vi "call service _ get time.vi"(7 "error in (no error)":errorcluster, 10 "TCP Network Connection in":refnum<k5>) -> (0 "error out":errorcluster, 2 "value":T1, 3 "TCP Network Connection out":refnum<k5>)   [LabVIEW 2015]
uses:
  <vilib>/MediaMongrels Ltd/WebSockets/WebSockets/WebSockets.lvlib
panel:
  in  "ros call service ctl.":T1
  out "Data":string
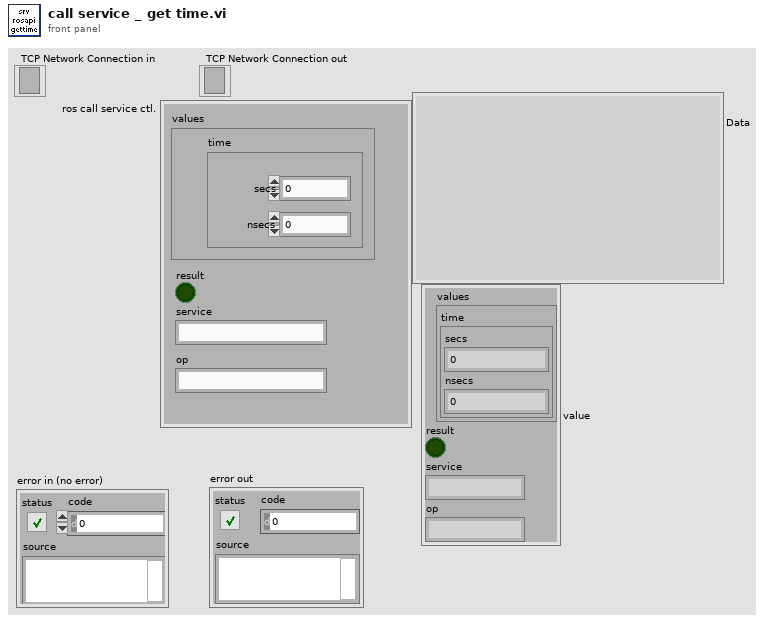
[diagram p1: front panel]
types:
  T1 = cluster{"values":cluster{"time":cluster{"secs":dbl, "nsecs":dbl}}, "result":bool, "service":string, "op":string}
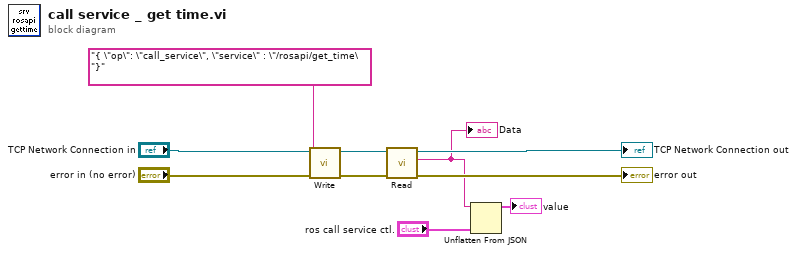
[diagram p0: block diagram]
diagram:
  n1 = call <vilib>:"Write.vi"("error in (no error)"="error in (no error)", "Data"="{ \"op\": \"call_service\", \"service\" : \"/rosapi/get_time\"}", "WebSocket Connection in"="TCP Network Connection in") -> ("error out"=w7:errorcluster, "WebSocket Connection out"=w6:refnum<k5>)  [unwired: 7 in]
  n2 = call <vilib>:"Read.vi"("error in (no error)"=w7, "WebSocket Connection in"=w6) -> ("error out"=→"error out":errorcluster, "Data"=w3:string, "WebSocket Connection out"=→"TCP Network Connection out":refnum<k5>)  [unwired: 6 in, 1 out]
  "Data" <- w3
  n3 = Unflatten From JSON(JSON string=w3, type and defaults="ros call service ctl.") -> (value=→"value":T1)  [unwired: 5 in, 1 out]
